vi "get index type definitions.vi"(10 "channel classification":T1, 11 "fixed channel configuration in":refnum<class "user control module configuration.lvclass">) -> (1 "valid?":bool, 2 "index cluster":variant, 3 "fixed channel configuration out":refnum<class "user control module configuration.lvclass">)   [LabVIEW 2013, in "user control module configuration.lvclass"]
uses:
  user control module configuration.lvclass
  <vilib>/NI/Tag Bus Module Framework/channel/channel classification.ctl
  input data indices.ctl
  output data indices.ctl
  parameter data indices.ctl
  result data indices.ctl
  <vilib>/NI/Tag Bus Module Framework/channel/TBM channel.lvclass
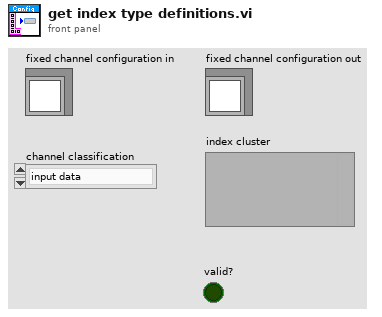
[diagram p1: front panel]
types:
  T1 = typedef "TBM channel.lvclass/channel classification.ctl" = enum16{"input data", "output data", "processing parameter", "processing result"}
  T2 = typedef "user control module configuration.lvclass/input data indices.ctl" = cluster{"Single.placeholder":i32}
  T3 = typedef "user control module configuration.lvclass/output data indices.ctl" = cluster{"Single.placeholder":i32}
  T4 = typedef "user control module configuration.lvclass/parameter data indices.ctl" = cluster{"Single.placeholder":i32}
  T5 = typedef "user control module configuration.lvclass/result data indices.ctl" = cluster{"Single.placeholder":i32}
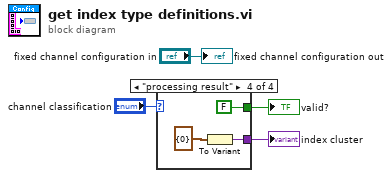
[diagram p0: block diagram]
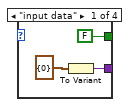
[diagram p2: hidden frame]
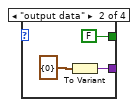
[diagram p3: hidden frame]
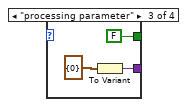
[diagram p4: hidden frame]
diagram:
  n1 = case shown="\"processing result\"" "channel classification" {
    tunnel: [w6 w10 w13 w16] -> w2
    tunnel: [FALSE FALSE FALSE FALSE] -> w1
    frame "input data" {
      n2 = To Variant(anything=T2 {"Single.placeholder"=0} ("Cluster")) -> (Variant=w6:variant)
    }
    frame "output data" {
      n3 = To Variant(anything=T3 {"Single.placeholder"=0} ("Cluster")) -> (Variant=w10:variant)
    }
    frame "processing parameter" {
      n4 = To Variant(anything=T4 {"Single.placeholder"=0} ("Cluster")) -> (Variant=w13:variant)
    }
    frame "processing result" {
      n5 = To Variant(anything=T5 {"Single.placeholder"=0} ("Cluster")) -> (Variant=w16:variant)
    }
  }
  "index cluster" <- w2
  "valid?" <- w1
  "fixed channel configuration out" <- "fixed channel configuration in"
